vi "event pair -- create.vi"(0 "talkto":T2, 5 "talkback":T1) -> (8 "even pair out":T3, 10 "takto event out":refnum<user-event>, 15 "talkback event out":refnum<user-event>)   [LabVIEW 2020]
uses:
  server talk-to-back pair.ctl
  server talkback message type.ctl
  server talkto message type.ctl
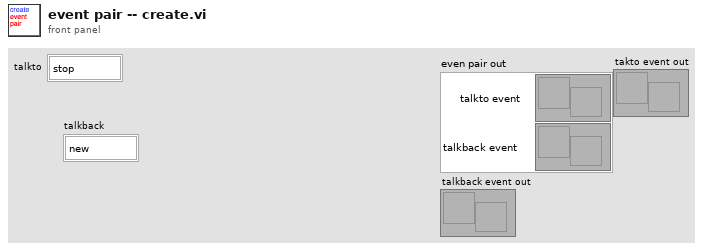
[diagram p1: front panel]
types:
  T1 = typedef "server talkback message type.ctl" = cluster{"message":enum16{"new", "void"}}
  T2 = typedef "server talkto message type.ctl" = cluster{"message":enum16{"stop", "start", "update pars", "update request", "new", "launch", "exit", "get", "reset", "pause", "unpause"}}
  T3 = typedef "server talk-to-back pair.ctl" = cluster{"talkback event":refnum<user-event>, "talkto event":refnum<user-event>}
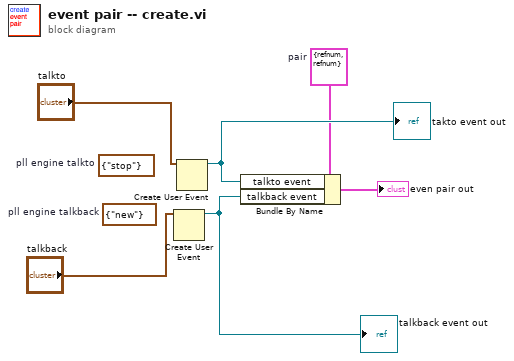
[diagram p0: block diagram]
diagram:
  w4 = T3 {"talkback event"=refnum, "talkto event"=refnum}  # pair
  (unwired) T1 {"message"=enum."new"}  # pll engine talkback
  (unwired) T2 {"message"=enum."stop"}  # pll engine talkto
  n1 = Create User Event(user event datatype="talkback") -> (user event=w6:refnum<user-event>)  [unwired: 1 in, 1 out]
  "talkback event out" <- w6
  n2 = Create User Event(user event datatype="talkto") -> (user event=w5:refnum<user-event>)  [unwired: 1 in, 1 out]
  "takto event out" <- w5
  n3 = Bundle By Name(cluster=w4, "talkto event"=w5, "talkback event"=w6) -> (→"even pair out":T3)
